vi "lv get display name.vi"(8 "error in (no error)":errorcluster, 11 "client handle":i32) -> (0 "error out":errorcluster, 3 "outbuffer":string)   [LabVIEW 2026]
uses:
  bin/nominalClient_64.dll
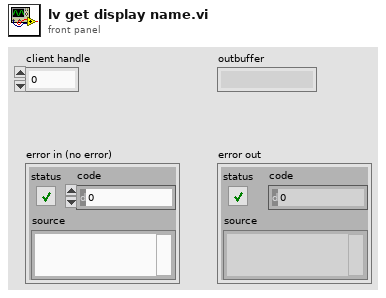
[diagram p1: front panel]
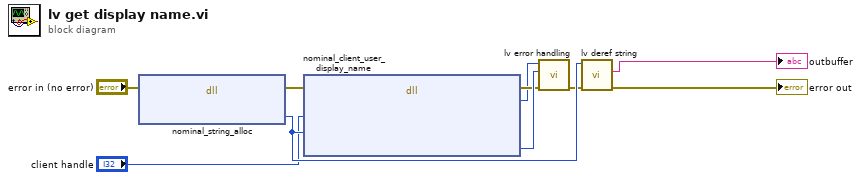
[diagram p0: block diagram]
diagram:
  n1 = dll-call lib="C:/sw/nominal-c/bin/nominalClient_64.dll" fn="nominal_string_alloc"(error in="error in (no error)") -> (error out=w2:errorcluster, "string handle"=w9:i32)  [unwired: 4 in, 1 out]
  n2 = dll-call lib="C:/sw/nominal-c/bin/nominalClient_64.dll" fn="nominal_client_user_display_name"(error in=w2, "client handle"="client handle", "display name handle"=w9) -> (error out=w7:errorcluster, "return type"=w6:i32, "errorout"=w10:u64)  [unwired: 5 in, 1 out]
  n3 = call "lv error handling.vi"("error in"=w7, "error handle"=w10, "return code"=w6) -> ("error out"=w8:errorcluster)  [unwired: 8 in]
  n4 = call "lv deref string.vi"("error in"=w8, "string handle"=w9) -> ("error out"=→"error out":errorcluster, "outbuffer"=→"outbuffer":string)  [unwired: 8 in]
